vi "notes_subVI.vi"(7 "previous notes":string) -> (8 "notes to add":string)   [LabVIEW 2014]
panel:
  in  "Add notes to experiment file. Do not use \"enter\" key to skip lines.":string
  in  "ok":bool
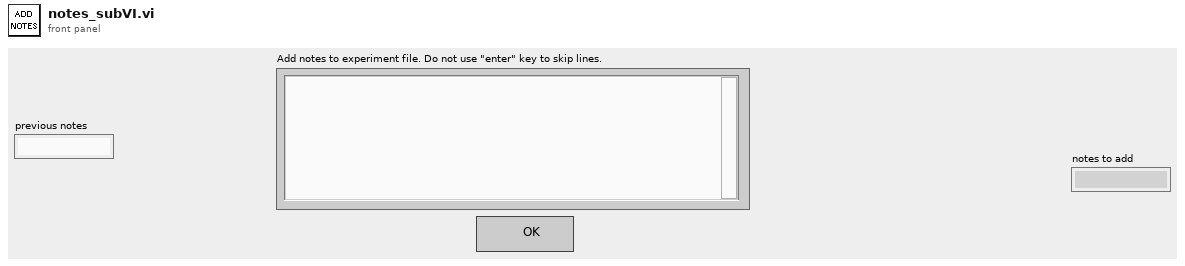
[diagram p1: front panel]
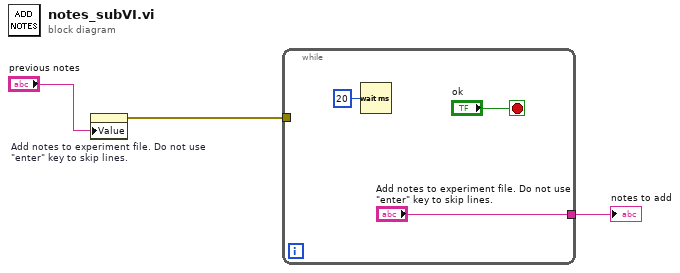
[diagram p0: block diagram]
diagram:
  n1 = property on="Add notes to experiment file. Do not use \"enter\" key to skip lines." class="Str"("Value"="previous notes") -> (error out=w1:errorcluster)  [unwired: 2 in, 1 out]
  n2 = while {
    tunnel: ["Add notes to experiment file. Do not use \"enter\" key to skip lines."] -> w3
    tunnel: w1 -> [_]
    stop <- "ok" stop-if-true
    n3 = Wait (ms)(milliseconds to wait=u32 20) -> ()  [unwired: 1 out]
  }
  "notes to add" <- w3
